vi "MultiSelect.vi"() -> ()   [LabVIEW 2011]
panel:
  in  "stop":bool
  out "Selected":i32(listbox)
  in  "MultiSelect":i32[](listbox)
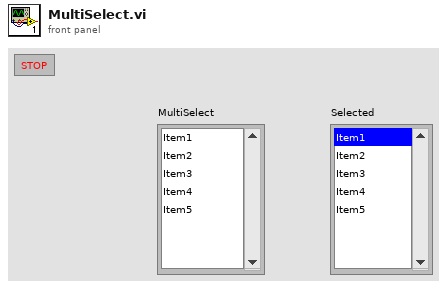
[diagram p1: front panel]
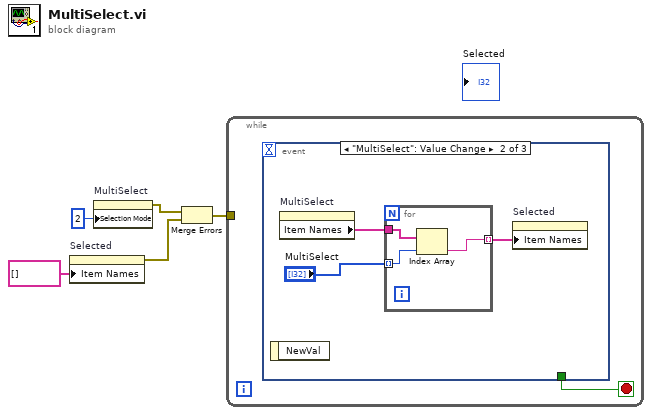
[diagram p0: block diagram]
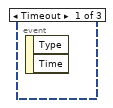
[diagram p2: hidden frame]
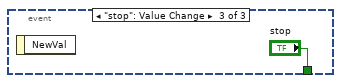
[diagram p3: hidden frame]
diagram:
  n1 = property on="Selected" class="LstBox (strict)"("Item Names"=string[] []) -> (error out=w2:errorcluster)  [unwired: 2 in, 1 out]
  n2 = property on="MultiSelect" class="LstBox (strict)"("Selection Mode"=2) -> (error out=w3:errorcluster)  [unwired: 2 in, 1 out]
  n3 = Merge Errors(w3, w2) -> (w1:errorcluster)
  n4 = while {
    tunnel: w1 -> [_]
    stop <- w6 stop-if-true
    n5 = event shown="[1] \"MultiSelect\": Value Change" {
      selector: _ -> [_ _ _]
      dyn-events: _ -> [_ _ _]
      timeout: _ -> [_ _ _]
      tunnel: [_ _ "stop"] -> w6
      event Timeout {
        n6 = event-data() -> ()  [unwired: 1 in, 2 out]
      }
      event "MultiSelect": Value Change {
        n7 = event-data() -> ()  [unwired: 1 in, 1 out]
        n8 = property on="MultiSelect" class="LstBox (strict)"() -> ("Item Names"=w9:string[])  [unwired: 2 in, 2 out]
        n9 = for {
          tunnel: w9 -> [w12]
          tunnel: "MultiSelect" -> [w11] mode=indexing
          tunnel: [w10] -> w7 mode=indexing
          n10 = Index Array(array=w12, index=w11) -> (element=w10:string)
        }
        n11 = property on="Selected" class="LstBox (strict)"("Item Names"=w7) -> ()  [unwired: 2 in, 2 out]
      }
      event "stop": Value Change {
        n12 = event-data() -> ()  [unwired: 1 in, 1 out]
      }
    }
  }
